vi "As Minimal Cluster Array.vi"(8 "error in (no error)":errorcluster, 11 "Controller Array in":refnum<class "Controller Array.lvclass">) -> (0 "error out":errorcluster, 2 "Controller Array":T1, 3 "Controller Array out":refnum<class "Controller Array.lvclass">)   [LabVIEW 2020, in "Controller Array.lvclass"]
uses:
  Controller Array.lvclass
  Minimal Controller Cluster Array.ctl
  Controller/Minimal Controller Cluster.ctl
  Controller Array.lvclass/Controller Array.ctl
  Controller/Generic Plugin.lvclass
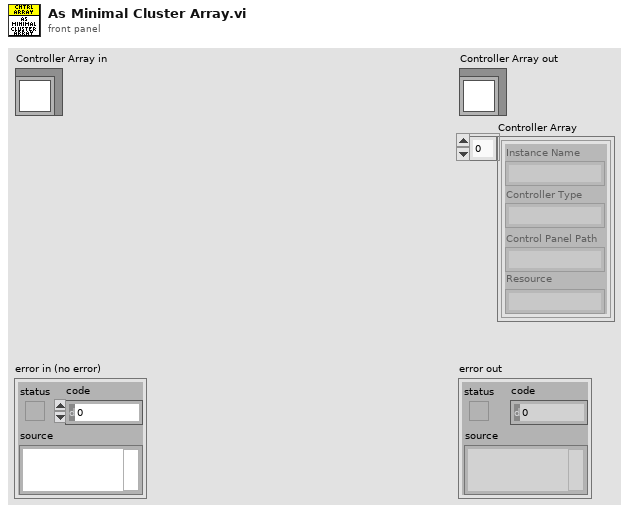
[diagram p1: front panel]
types:
  T1 = typedef "Generic Plugin.lvclass/Minimal Controller Cluster Array.ctl" = T2[]
  T2 = typedef "Generic Plugin.lvclass/Minimal Controller Cluster.ctl" = cluster{"Instance Name":string, "Controller Type":string, "Control Panel Path":string, "Resource":string}
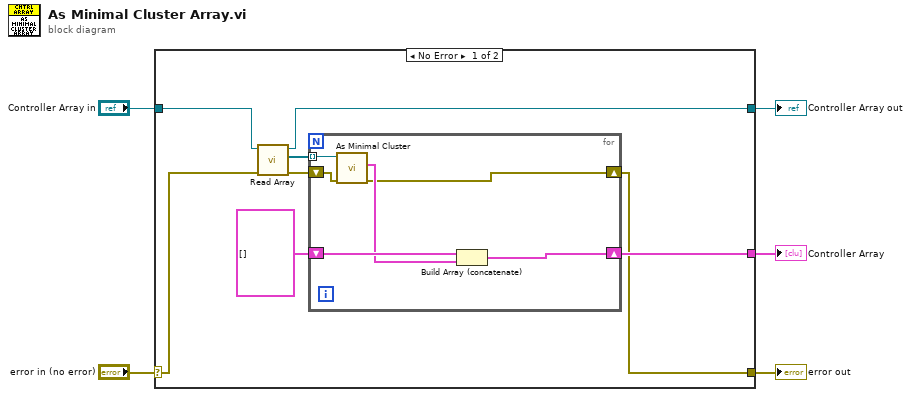
[diagram p0: block diagram]
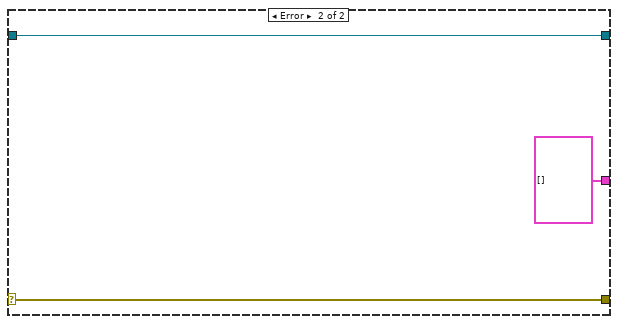
[diagram p2: hidden frame]
diagram:
  n1 = case shown="No Error" "error in (no error)" {
    selector: "error in (no error)" -> [w9 w22]
    tunnel: [w6 w22] -> w4
    tunnel: [w11 w21] -> w2
    tunnel: "Controller Array in" -> [w10 w21]
    tunnel: [w7 T1 []] -> w1
    frame No Error {
      n2 = call "Read Array.vi"("error in (no error)"=w9, "Controller Array in"=w10) -> ("error out"=w8:errorcluster, "Array"=w13:refnum<class "Generic Plugin.lvclass">[], "Controller Array out"=w11:refnum<class "Controller Array.lvclass">)  [unwired: 7 in]
      n3 = for {
        tunnel: w13 -> [w19] mode=indexing
        shift-right: [w17] -> w7
        shift-left: T1 [] -> [w18]
        shift-right: [w14] -> w6
        shift-left: w8 -> [w15]
        n4 = call-dynamic "As Minimal Cluster.vi"("error in (no error)"=w15, "Generic Controller in"=w19) -> ("error out"=w14:errorcluster, "Minimal Cluster out"=w16:T2)  [unwired: 7 in, 1 out]
        n5 = Build Array (concatenate)(w18, w16) -> (w17:T1)
      }
    }
    frame Error {
    }
  }
  "error out" <- w4
  "Controller Array out" <- w2
  "Controller Array" <- w1
